vi "readPumpSpeed.vi"(8 "error in (no error)":errorcluster, 11 "Pump.Simulated in":refnum<class "Pump.Simulated.lvclass">) -> (0 "error out":errorcluster, 2 "Pump Speed":dbl, 3 "Pump.Simulated out":refnum<class "Pump.Simulated.lvclass">)   [LabVIEW 2014, in "Pump.Simulated.lvclass"]
uses:
  Pump.Simulated.lvclass
  Pump.Simulated.lvclass/Pump.Simulated.ctl
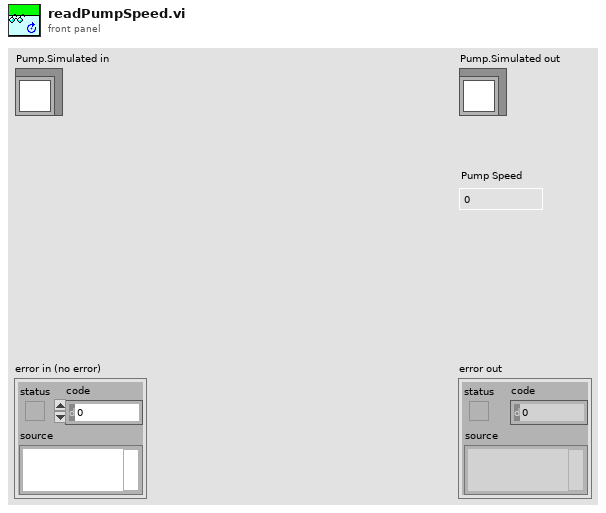
[diagram p1: front panel]
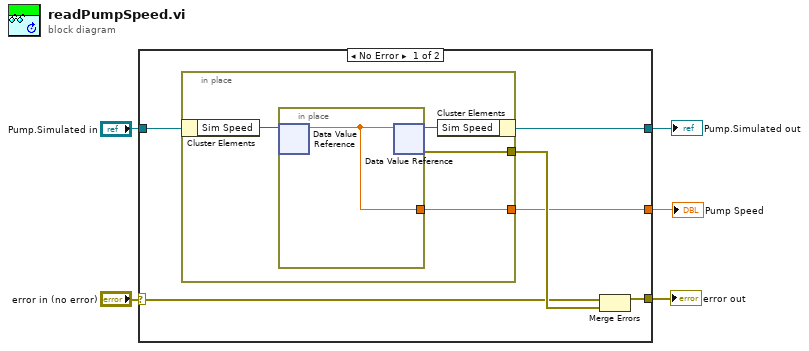
[diagram p0: block diagram]
diagram:
  n1 = case shown="No Error" "error in (no error)" {
    selector: "error in (no error)" -> [w6 w18]
    tunnel: [w9 w18] -> w1
    tunnel: [w11 w17] -> w2
    tunnel: "Pump.Simulated in" -> [w7 w17]
    tunnel: [w8 _] -> w5
    frame No Error {
      n2 = in-place {
        in-place-border: [w12] -> w10
        in-place-border: [w13] -> w8
        n3 = in-place-cluster #1(w7) -> ("Sim Speed"=w15:refnum<data-value>)
        n4 = in-place {
          in-place-border: [w16] -> w13
          n5 = in-place-dvr #2(w15) -> (w16:dbl)  [unwired: 1 out]
          n6 = in-place-dvr #2(w16) -> (w14:refnum<data-value>, w12:errorcluster)
        }
        n7 = in-place-cluster #1("Sim Speed"=w14) -> (w11:refnum<class "Pump.Simulated.lvclass">)
      }
      n8 = Merge Errors(w6, w10) -> (w9:errorcluster)
    }
    frame Error {
    }
  }
  "error out" <- w1
  "Pump.Simulated out" <- w2
  "Pump Speed" <- w5
